vi "Flush Object Buffer.vi"(8 "error in":errorcluster, 11 "Buffer in":refnum<data-value>) -> (0 "error out":errorcluster, 2 "elements":refnum<class>[](array[class]), 3 "Buffer":refnum<data-value>)   [LabVIEW 2013, in "CircularBuffer.lvlib" / "ObjectBuffer.lvclass"]
doc: "This VI returns data from the ring buffer starting from the oldest data and ending with the newest.\n\nThe data is duplicated at the output so this VI allocates new place in the memory for the output."
uses:
  ObjectBuffer.lvclass
  VariantBuffer/VariantBuffer.lvclass
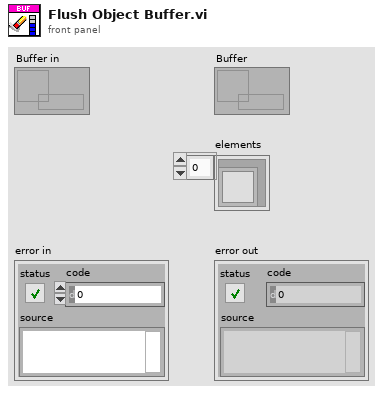
[diagram p1: front panel]
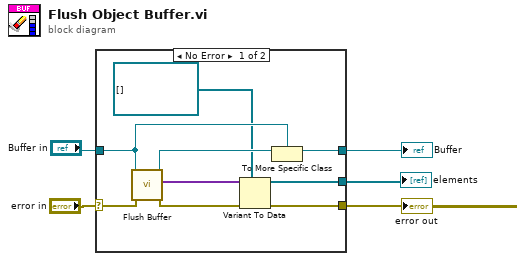
[diagram p0: block diagram]
diagram:
  n1 = case shown="No Error" "error in" {
    selector: "error in" -> [w14 w15]
    tunnel: "Buffer in" -> [w7 w16]
    tunnel: [w8 w16] -> w2
    tunnel: [w12 w15] -> w4
    tunnel: [w10 _] -> w1
    frame No Error {
      n2 = call "Flush Buffer.vi"("error in"=w14, "Buffer in"=w7) -> ("error out"=w13:errorcluster, "elements"=w11:variant[], "Buffer"=w9:refnum<data-value>)  [unwired: 7 in]
      n3 = Variant To Data(error in=w13, type=refnum<class>[] [] ("elements"), Variant=w11) -> (data=w10:refnum<class>[], error out=w12:errorcluster)
      n4 = To More Specific Class(target class=w7, reference=w9) -> (specific class reference=w8:refnum<data-value>)  [unwired: 1 in, 1 out]
    }
    frame Error {
    }
  }
  "error out" <- w4
  "Buffer" <- w2
  "elements" <- w1
